vi "fgv_AO_DAQmx-Config.vi"(7 "cmd":T2, 8 "error in":errorcluster, 11 "9269 AO Config":T1={"Ch"="cDAQ1Mod1/ao0", "Max V"=5.0, "Min V"=-5.0, " Rate"=1000.0, "N pts"=100, "sample mode"=10178} {"sample mode" items=["유한 샘플"=10178, "연속 샘플"=10123, "하드웨어 타이밍에 의한 단일 포인트"=12522]}) -> (0 "error out":errorcluster, 3 "config 2":T1={"Ch"="cDAQ1Mod1/ao0", "Max V"=5.0, "Min V"=-5.0, " Rate"=1000.0, "N pts"=100, "sample mode"=10178} {"sample mode" items=["유한 샘플"=10178, "연속 샘플"=10123, "하드웨어 타이밍에 의한 단일 포인트"=12522]})   [LabVIEW 2019]
uses:
  _ctrl/rw.ctl
  _ctrl/cDAQ-9269 Config.ctl
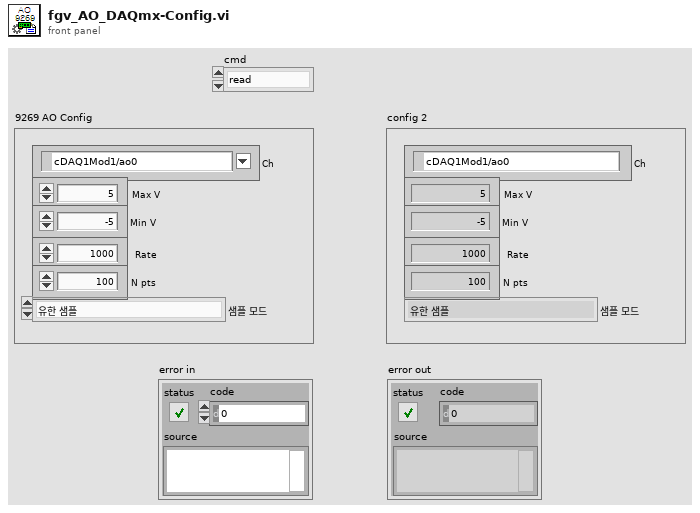
[diagram p1: front panel]
types:
  T1 = typedef "cDAQ-9269 Config.ctl" = cluster{"Ch":tag, "Max V":dbl, "Min V":dbl, " Rate":dbl, "N pts":i32, "sample mode":i32}
  T2 = typedef "rw.ctl" = enum16{"read", "write"}
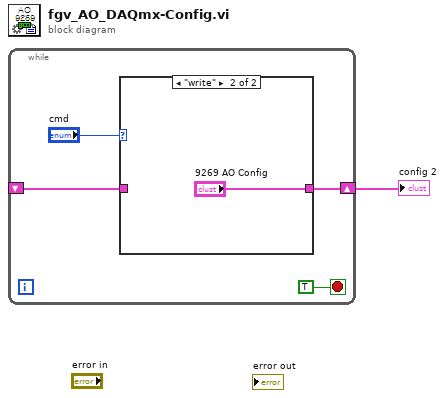
[diagram p0: block diagram]
diagram:
  n1 = while {
    shift-right: [w3] -> w1
    shift-left: _ -> [w2]
    stop <- TRUE stop-if-true
    n2 = case shown="\"write\"" "cmd" {
      tunnel: [w6 "9269 AO Config"] -> w3
      tunnel: w2 -> [w6 _]
      frame "read", Default {
      }
      frame "write" {
      }
    }
  }
  "config 2" <- w1
